vi "TRITON_TCP_COMS.vi"() -> (0 "Cluster":T1)   [LabVIEW 2015]
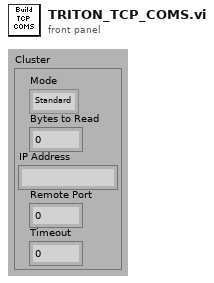
[diagram p1: front panel]
types:
  T1 = cluster{"Mode":enum16{"Standard", "Buffered", "CRLF", "Immediate"}, "Bytes to Read":i32, "IP Address":string, "Remote Port":i32, "Timeout":i32}
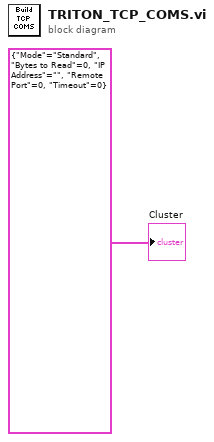
[diagram p0: block diagram]
diagram:
  "Cluster" <- T1 {"Mode"=enum."Standard", "Bytes to Read"=0, "IP Address"="", "Remote Port"=0, "Timeout"=0}
